vi "VeriStand DSF.Transfer.Configuration.Create.vi"(8 "error in (no error)":errorcluster, 10 "Section Ref":T1=18446744073709551615 format="%.0x", 11 "Device Ref":T1=18446744073709551615 format="%.0x") -> (0 "error out":errorcluster, 3 "Transfer Configuration":refnum<class "VeriStand DSF.Transfer.Configuration.lvclass">)   [LabVIEW 2017, in "Data Sharing Custom Device Engine.lvlib" / "VeriStand DSF.Transfer.Configuration.lvclass"]
uses:
  VeriStand DSF.Transfer.Configuration.lvclass
  <vilib>/NI Veristand/Custom Device API/Custom Device Item Ref.ctl
  VeriStand DSF.Transfer.Configuration.lvclass/VeriStand DSF.Transfer.Configuration.ctl
  <vilib>/NI Veristand/Custom Device API/Custom Device API.lvlib
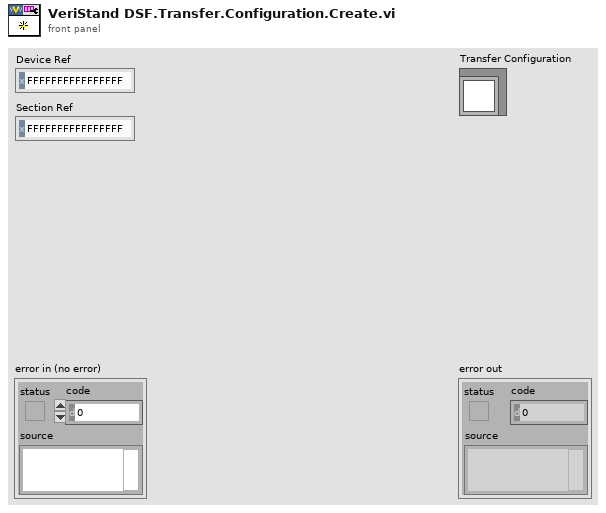
[diagram p1: front panel]
types:
  T1 = typedef "Custom Device API.lvlib/Custom Device Item Ref.ctl" = u64
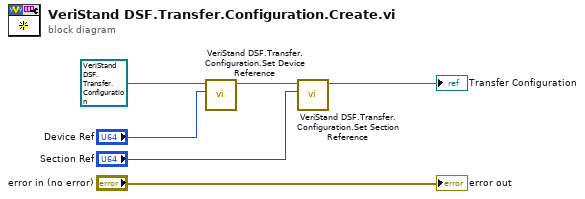
[diagram p0: block diagram]
diagram:
  n1 = call "VeriStand DSF.Transfer.Configuration.Set Device Reference.vi"("Device Reference"="Device Ref", "VeriStand DSF.Transfer.Configuration in"=refnum<class "VeriStand DSF.Transfer.Configuration.lvclass"> refnum ("Transfer Configuration")) -> ("VeriStand DSF.Transfer.Configuration out"=w4:refnum<class "VeriStand DSF.Transfer.Configuration.lvclass">)  [unwired: 9 in]
  n2 = call "VeriStand DSF.Transfer.Configuration.Set Section Reference.vi"("Section Ref"="Section Ref", "VeriStand DSF.Transfer.Configuration in"=w4) -> ("VeriStand DSF.Transfer.Configuration out"=→"Transfer Configuration":refnum<class "VeriStand DSF.Transfer.Configuration.lvclass">)  [unwired: 9 in]
  "error out" <- "error in (no error)"
